vi "math2.vi"(9 "valori_tutti":dbl[][](array[numeric])) -> (0 "incertezza":dbl[](array[numeric]), 2 "media":dbl[](array[numeric]))   [LabVIEW 2021]
uses:
  <vilib>/Analysis/baseanly.llb/Mean (DBL).vi
  <vilib>/Analysis/NI_AALBase.lvlib
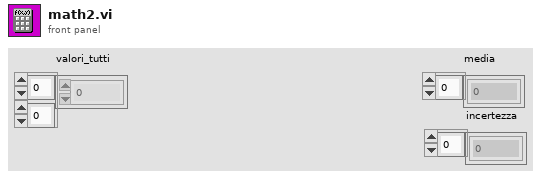
[diagram p1: front panel]
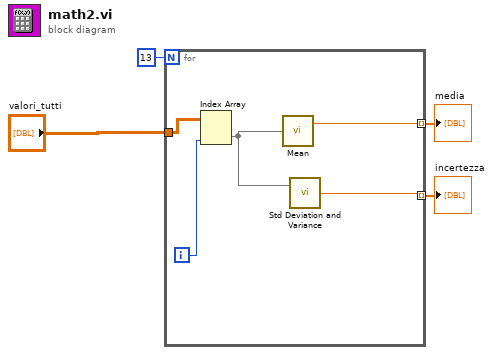
[diagram p0: block diagram]
diagram:
  n1 = for {
    N: 13 -> [_]
    tunnel: [w8] -> w2 mode=indexing
    tunnel: [w6] -> w1 mode=indexing
    tunnel: "valori_tutti" -> [w5]
    i -> [w9]
    n2 = Index Array(array=w5, index (col)=w9) -> (element=w7:dbl[])  [unwired: 1 in]
    n3 = call-poly <vilib>:"Mean.vi"("X"=w7) -> ("mean"=w8:dbl)  [unwired: 1 out]
    n4 = call <vilib>:"Std Deviation and Variance.vi"("X"=w7) -> ("standard deviation"=w6:dbl)  [unwired: 1 in, 2 out]
  }
  "media" <- w2
  "incertezza" <- w1
